vi "ArmBackward.vi"(10 "BackwardLimitSwitch":T1) -> (2 "Done?":bool)   [LabVIEW 2012]
uses:
  <vilib>/Rock Robotics/WPI/DigitalInput/WPI_DigitalInputDevRef.ctl
  <vilib>/Rock Robotics/SystemInterfaces/DIO/FPGA_DIOChannel.ctl
  <vilib>/Rock Robotics/SystemInterfaces/Typedef/FPGA_TypedefDigitalModule.ctl
  Robot Global Data.vi
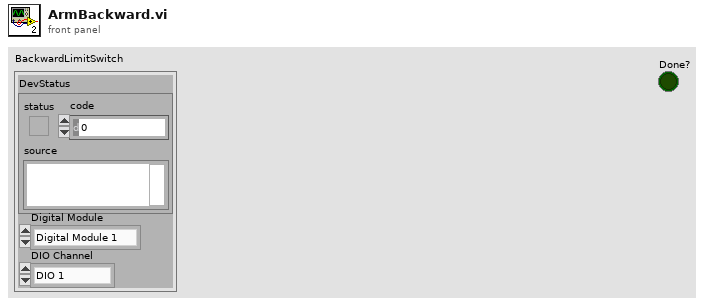
[diagram p1: front panel]
types:
  T1 = typedef "WPI_DigitalInputDevRef.ctl" = cluster{"DevStatus":errorcluster, "DIO Channel":T2, "Digital Module":T3}
  T2 = typedef "FPGA_DIOChannel.ctl" = enum8{"DIO 1", "DIO 2", "DIO 3", "DIO 4", "DIO 5", "DIO 6", "DIO 7", "DIO 8", "DIO 9", "DIO 10", "DIO 11", "DIO 12", "DIO 13", "DIO 14", "Invalid"}
  T3 = typedef "FPGA_TypedefDigitalModule.ctl" = enum16{"Digital Module 1", "Digital Module 2"}
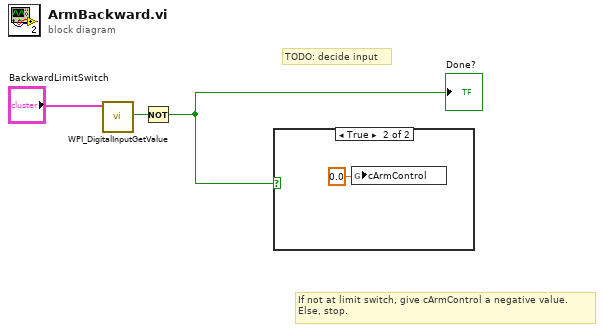
[diagram p0: block diagram]
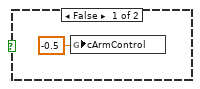
[diagram p2: hidden frame]
diagram:
  # "If not at limit switch, give cArmControl a negative value.\nElse, stop."
  # "TODO: decide input"
  n1 = call <vilib>:"WPI_DigitalInputGetValue.vi"("DigitalInputDevRef"="BackwardLimitSwitch") -> ("Value"=w3:bool)  [unwired: 8 in, 2 out]
  n2 = Not(x=w3) -> (.not. x?=w1:bool)
  "Done?" <- w1
  n3 = case shown="True" w1 {
    frame False {
      n4 = global write "Robot Global Data.vi" "cArmControl"(-0.5 ("Output")) -> ()
    }
    frame True {
      n5 = global write "Robot Global Data.vi" "cArmControl"(0.0 ("Output")) -> ()
    }
  }
